vi "TxRx.vi"(4 "Timeout":u32=1000 format="%.0f ms", 6 "WaitBeforeReply":u32=100 format="%.0f ms", 7 "comport in":refnum<visa-resource-name>, 8 "error in":errorcluster, 9 "Expected Reply Length":i32=-1, 10 "ReplyFirstByte":T1 items=["ANALOG_IO_MESSAGE"=224, "DIGITAL_IO_MESSAGE"=144, "REPORT_ANALOG_PIN"=192, "REPORT_DIGITAL_PORT"=208, "START_SYSEX"=240, "END_SYSEX"=247, "SET_PIN_MODE"=244, "SET_DIGITAL_PIN_VALUE"=245, "PROTOCOL_VERSION"=249, "SYSTEM_RESET"=255, "SYSEX.EXTENDED_ID"=0, "SYSEX.RESERVED_USER_COMMANDs"=1, "SYSEX.ANALOG_MAPPING_QUERY"=105, "SYSEX.ANALOG_MAPPING_RESPONSE"=106, "SYSEX.CAPABILITY_QUERY"=107, "SYSEX.CAPABILITY_RESPONSE"=108, "SYSEX.PIN_STATE_QUERY"=109, "SYSEX.PIN_STATE_RESPONSE"=110, "SYSEX.REPORT_FIRMWARE"=121, "SYSEX.EXTENDED_ANALOG"=111, "SYSEX.STRING_DATA"=113, "SYSEX.REALTIME"=127, "SYSEX.NON_REALTIME"=126, "SYSEX.SAMPLING_INTERVAL"=122], 11 "MessageToSend":u8[](array[numeric]) format="%x") -> (0 "error out":errorcluster={"status"=TRUE, "code"=5001, "source"="Communication Failed. \nDid not receive expected char   '00'"}, 1 "UnprocessedBytes":string, 2 "ReplyFirstByte out":T1 items=["ANALOG_IO_MESSAGE"=224, "DIGITAL_IO_MESSAGE"=144, "REPORT_ANALOG_PIN"=192, "REPORT_DIGITAL_PORT"=208, "START_SYSEX"=240, "END_SYSEX"=247, "SET_PIN_MODE"=244, "SET_DIGITAL_PIN_VALUE"=245, "PROTOCOL_VERSION"=249, "SYSTEM_RESET"=255, "SYSEX.EXTENDED_ID"=0, "SYSEX.RESERVED_USER_COMMANDs"=1, "SYSEX.ANALOG_MAPPING_QUERY"=105, "SYSEX.ANALOG_MAPPING_RESPONSE"=106, "SYSEX.CAPABILITY_QUERY"=107, "SYSEX.CAPABILITY_RESPONSE"=108, "SYSEX.PIN_STATE_QUERY"=109, "SYSEX.PIN_STATE_RESPONSE"=110, "SYSEX.REPORT_FIRMWARE"=121, "SYSEX.EXTENDED_ANALOG"=111, "SYSEX.STRING_DATA"=113, "SYSEX.REALTIME"=127, "SYSEX.NON_REALTIME"=126, "SYSEX.SAMPLING_INTERVAL"=122], 3 "ReceivedMessage":u8[](array[numeric]) format="%x", 5 "comport out":refnum<visa-resource-name>)   [LabVIEW 2020, in "FirmataClient.lvlib"]
doc: "Handles Transmission and Reception geared towards the Firmata Protocol"
uses:
  FirmataClient.lvlib
  controls/FirmataProtocolConstants.ctl
  <vilib>/regexp/Match Regular Expression.xnode
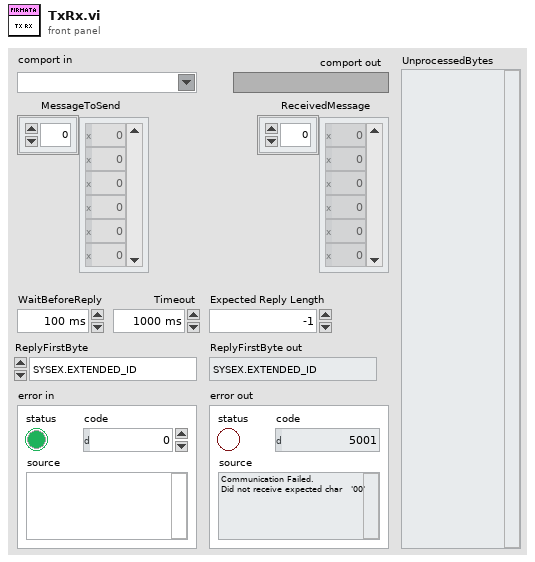
[diagram p1: front panel]
types:
  T1 = typedef "FirmataClient.lvlib/FirmataProtocolConstants.ctl" = u16
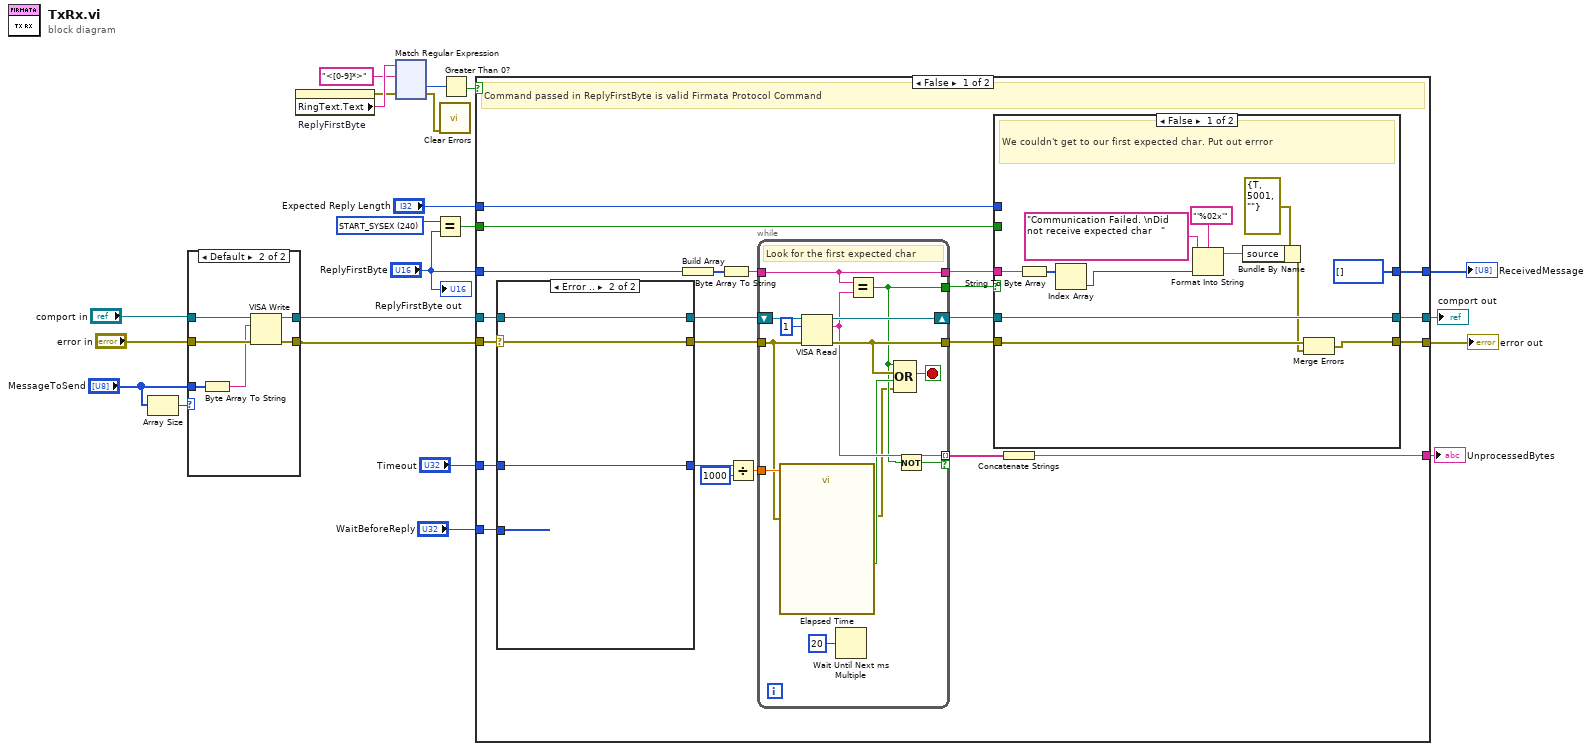
[diagram p0: block diagram]
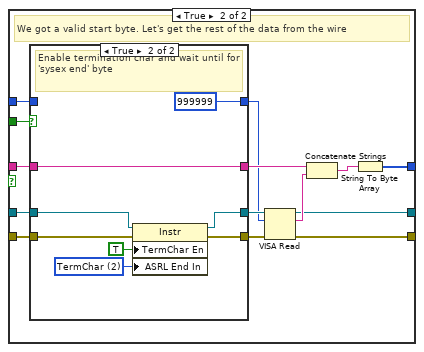
[diagram p2: hidden frame]
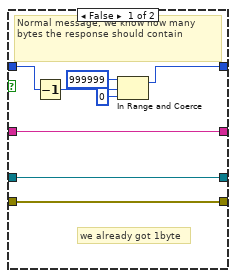
[diagram p3: hidden frame]
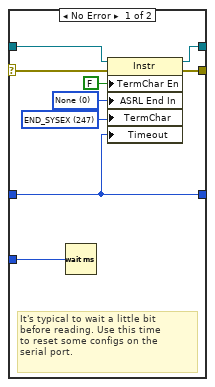
[diagram p4: hidden frame]
diagram:
  w14 = T1 240 items=["ANALOG_IO_MESSAGE"=224, "DIGITAL_IO_MESSAGE"=144, "REPORT_ANALOG_PIN"=192, "REPORT_DIGITAL_PORT"=208, "START_SYSEX"=240, "END_SYSEX"=247, "SET_PIN_MODE"=244, "SET_DIGITAL_PIN_VALUE"=245, "PROTOCOL_VERSION"=249, "SYSTEM_RESET"=255, "SYSEX.EXTENDED_ID"=0, "SYSEX.RESERVED_USER_COMMANDs"=1, "SYSEX.ANALOG_MAPPING_QUERY"=105, "SYSEX.ANALOG_MAPPING_RESPONSE"=106, "SYSEX.CAPABILITY_QUERY"=107, "SYSEX.CAPABILITY_RESPONSE"=108, "SYSEX.PIN_STATE_QUERY"=109, "SYSEX.PIN_STATE_RESPONSE"=110, "SYSEX.REPORT_FIRMWARE"=121, "SYSEX.EXTENDED_ANALOG"=111, "SYSEX.STRING_DATA"=113, "SYSEX.REALTIME"=127, "SYSEX.NON_REALTIME"=126, "SYSEX.SAMPLING_INTERVAL"=122] ("ReplyFirstByte")
  n1 = Array Size(array="MessageToSend") -> (size(s)=w17:i32)
  n2 = case shown="Default" w17 {
    tunnel: "error in" -> [w23 w30]
    tunnel: "comport in" -> [w24 w29]
    tunnel: [w24 w28] -> w20
    tunnel: "MessageToSend" -> [_ w27]
    tunnel: [w23 w25] -> w19
    frame 0 {
    }
    frame Default {
      n3 = Byte Array To String(unsigned byte array=w27) -> (string=w26:string)
      n4 = VISA Write(VISA resource name=w29, write buffer=w26, error in (no error)=w30) -> (VISA resource name out=w28:refnum<visa-resource-name>, error out=w25:errorcluster)  [unwired: 1 out]
    }
  }
  n5 = property on="ReplyFirstByte" class="Ring (strict)"() -> (error out=w2:errorcluster, "RingText.Text"=w12:string)  [unwired: 2 in, 1 out]
  n6 = xnode "Match Regular Expression"("input string"=w12, "regular expression"="<[0-9]*>", "error in"=w2) -> ("offset past match"=w10:i32, "error out"=w1:errorcluster)  [unwired: 3 in, 3 out]
  n7 = Equal?(x=w14, y="ReplyFirstByte") -> (x = y?=w13:bool)
  n8 = call <vilib>:"Clear Errors.vi"("error in (no error)"=w1) -> ()  [unwired: 5 in, 2 out]
  n9 = Greater Than 0?(x=w10) -> (x > 0?=w9:bool)
  n10 = case shown="False" w9 {
    tunnel: [w38 w123] -> w21
    tunnel: w20 -> [w51 w122]
    tunnel: w19 -> [w52 w123]
    tunnel: "Timeout" -> [w35 _]
    tunnel: "WaitBeforeReply" -> [w53 _]
    tunnel: w13 -> [w40 _]
    tunnel: "ReplyFirstByte" -> [w44 _]
    tunnel: [w37 _] -> w7
    tunnel: [w33 _] -> w6
    tunnel: [w32 w122] -> w4
    tunnel: "Expected Reply Length" -> [w31 _]
    frame False {
      # "Command passed in ReplyFirstByte is valid Firmata Protocol Command"
      n11 = case shown="Error .." w52 {
        selector: w52 -> [w115 w120]
        tunnel: [w114 w120] -> w50
        tunnel: w53 -> [w118 _]
        tunnel: [w113 w121] -> w49
        tunnel: w51 -> [w112 w121]
        tunnel: [w111 w119] -> w36
        tunnel: w35 -> [w111 w119]
        frame No Error {
          w110 = T1 247 items=["ANALOG_IO_MESSAGE"=224, "DIGITAL_IO_MESSAGE"=144, "REPORT_ANALOG_PIN"=192, "REPORT_DIGITAL_PORT"=208, "START_SYSEX"=240, "END_SYSEX"=247, "SET_PIN_MODE"=244, "SET_DIGITAL_PIN_VALUE"=245, "PROTOCOL_VERSION"=249, "SYSTEM_RESET"=255, "SYSEX.EXTENDED_ID"=0, "SYSEX.RESERVED_USER_COMMANDs"=1, "SYSEX.ANALOG_MAPPING_QUERY"=105, "SYSEX.ANALOG_MAPPING_RESPONSE"=106, "SYSEX.CAPABILITY_QUERY"=107, "SYSEX.CAPABILITY_RESPONSE"=108, "SYSEX.PIN_STATE_QUERY"=109, "SYSEX.PIN_STATE_RESPONSE"=110, "SYSEX.REPORT_FIRMWARE"=121, "SYSEX.EXTENDED_ANALOG"=111, "SYSEX.STRING_DATA"=113, "SYSEX.REALTIME"=127, "SYSEX.NON_REALTIME"=126, "SYSEX.SAMPLING_INTERVAL"=122] ("ReplyFirstByte")
          w117 = u16 0 items=["None", "Last Bit", "TermChar"] ("Serial Settings:End Mode for Reads")
          # "It's typical to wait a little bit\nbefore reading. Use this time\nto reset some configs on the \nserial port."
          n12 = Wait (ms)(milliseconds to wait=w118) -> ()  [unwired: 1 out]
          n13 = property class="Instr"(reference=w112, error in=w115, "TermChar En"=FALSE ("Message Based Settings:Termination Character Enable"), "ASRL End In"=w117, "TermChar"=w110, "Timeout"=w111) -> (reference out=w113:refnum<visa-resource-name>, error out=w114:errorcluster)
        }
        frame Error {
        }
      }
      n14 = Build Array(w44) -> (w48:T1[])
      n15 = Byte Array To String(unsigned byte array=w48) -> (string=w47:string)
      n16 = Divide(x=w36, y=u32 1000) -> (x/y=w46:dbl)
      n17 = while {
        tunnel: w50 -> [w97]
        shift-right: [w108] -> w42
        shift-left: w49 -> [w109]
        tunnel: [w106] -> w41
        tunnel: w47 -> [w102]
        tunnel: w46 -> [w104]
        tunnel: [w99] -> w43
        tunnel: [w102] -> w39
        tunnel: [w101] -> w34 mode=indexing if=w98
        stop <- w105 stop-if-true
        # "Look for the first expected char"
        n18 = call "Elapsed Time"("Time Target (s)"=w104, "error in (no error)"=w97) -> ("Time has Elapsed"=w100:bool, "error out"=w96:errorcluster)  [unwired: 10 in, 6 out]
        n19 = VISA Read(VISA resource name=w109, byte count=u32 1, error in (no error)=w97) -> (VISA resource name out=w108:refnum<visa-resource-name>, read buffer=w101:string, error out=w106:errorcluster)  [unwired: 1 out]
        n20 = Wait Until Next ms Multiple(millisecond multiple=u32 20) -> ()  [unwired: 1 out]
        n21 = Equal?(x=w102, y=w101) -> (x = y?=w99:bool)
        n22 = Compound Arithmetic op=OR(w99, w106, w100, w96) -> (w105:bool)
        n23 = Not(x=w99) -> (.not. x?=w98:bool)
      }
      n24 = case shown="False" w43 {
        tunnel: w42 -> [w58 w78]
        tunnel: [w55 w74] -> w38
        tunnel: w41 -> [w57 w79]
        tunnel: w40 -> [_ w77]
        tunnel: w39 -> [w65 w73]
        tunnel: [u8[] [] ("unsigned byte array") w67] -> w37
        tunnel: w31 -> [_ w70]
        tunnel: [w58 w66] -> w32
        frame False {
          # "We couldn't get to our first expected char. Put out errror"
          n25 = String To Byte Array(string=w65) -> (unsigned byte array=w63:u8[])
          n26 = Index Array(array=w63) -> (element=w61:u8)  [unwired: 1 in]
          n27 = Format Into String(format string="'%02x'", initial string="Communication Failed. \nDid not receive expected char   " ("source"), w61) -> (resulting string=w59:string)  [unwired: 1 in, 1 out]
          n28 = Bundle By Name(cluster=errorcluster {"status"=TRUE, "code"=5001, "source"=""} ("error out"), "source"=w59) -> (w54:errorcluster)
          n29 = Merge Errors(w57, w54) -> (w55:errorcluster)
        }
        frame True {
          # "We got a valid start byte. Let's get the rest of the data from the wire"
          n30 = case shown="True" w77 {
            tunnel: w79 -> [w86 w93]
            tunnel: [w86 w92] -> w76
            tunnel: w78 -> [w87 w91]
            tunnel: [w87 w90] -> w75
            tunnel: [w85 w89] -> w72
            tunnel: w73 -> [w85 w89]
            tunnel: [w82 u32 999999 ("byte count")] -> w69
            tunnel: w70 -> [w81 _]
            frame False {
              # "we already got 1byte"
              # "Normal message, we know how many bytes the response should contain"
              n31 = Decrement(x=w81) -> (x-1=w80:i32)
              n32 = In Range and Coerce(upper limit=u32 999999, x=w80, lower limit=u32 0) -> (coerced(x)=w82:u32)  [unwired: 1 out]
            }
            frame True {
              w95 = u16 2 items=["None", "Last Bit", "TermChar"] ("Serial Settings:End Mode for Reads")
              # "Enable termination char and wait until for 'sysex end' byte"
              n33 = property class="Instr"(reference=w91, error in=w93, "TermChar En"=TRUE ("Message Based Settings:Termination Character Enable"), "ASRL End In"=w95) -> (reference out=w90:refnum<visa-resource-name>, error out=w92:errorcluster)
            }
          }
          n34 = VISA Read(VISA resource name=w75, byte count=w69, error in (no error)=w76) -> (VISA resource name out=w66:refnum<visa-resource-name>, read buffer=w71:string, error out=w74:errorcluster)  [unwired: 1 out]
          n35 = Concatenate Strings(w72, w71) -> (w68:string)
          n36 = String To Byte Array(string=w68) -> (unsigned byte array=w67:u8[])
        }
      }
      n37 = Concatenate Strings(w34) -> (w33:string)
    }
    frame True {
      # "Unknown Command passed in ReplyFirstByte"
    }
  }
  "error out" <- w21
  "ReceivedMessage" <- w7
  "UnprocessedBytes" <- w6
  "comport out" <- w4
  "ReplyFirstByte out" <- "ReplyFirstByte"
